vi "Jump To Label.vi"(4 "error in (no error)":errorcluster, 5 "Loop Count (1)":i32=1 min=1 max=65535, 6 "Label  (1)":i32=1 min=1 max=100, 7 "VISA resource name":refnum<visa-resource-name>) -> (0 "error out":errorcluster, 3 "VISA resource name out":refnum<visa-resource-name>)   [LabVIEW 2018, in "Newport ESP301.lvlib"]
doc: "This command changes the flow of the program execution by jumping to a\npredefined label xx. This a flow control command that alters the normal sequential flow of a program. It must be used in conjunction with the DL command which defines a label.\nParameter Loop Count determines the number of times to repeat the jump before allowing the program to flow passed."
uses:
  Newport ESP301.lvlib
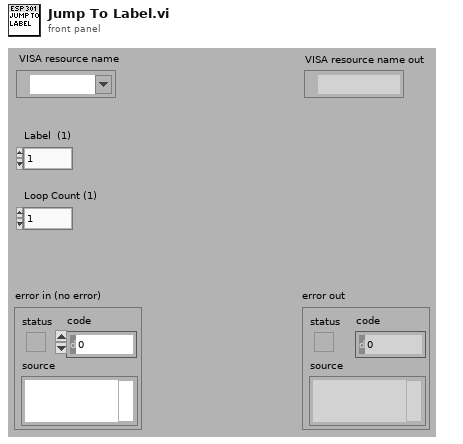
[diagram p1: front panel]
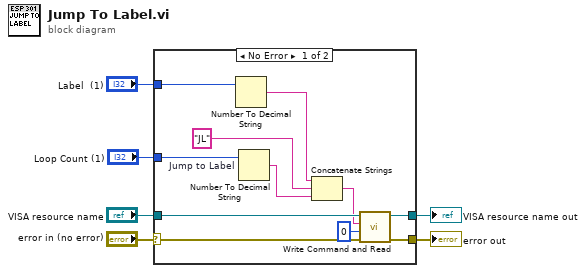
[diagram p0: block diagram]
diagram:
  n1 = case shown="No Error" "error in (no error)" {
    selector: "error in (no error)" -> [w16 w19]
    tunnel: [w15 w19] -> w6
    tunnel: "VISA resource name" -> [w17 w18]
    tunnel: [w14 w18] -> w5
    tunnel: "Label  (1)" -> [w11 _]
    tunnel: "Loop Count (1)" -> [w8 _]
    frame No Error {
      w12 = "JL"  # Jump to Label
      n2 = Number To Decimal String(number=w11) -> (decimal integer string=w13:string)  [unwired: 1 out]
      n3 = Number To Decimal String(number=w8) -> (decimal integer string=w7:string)  [unwired: 1 out]
      n4 = Concatenate Strings(w13, w12, w7) -> (w10:string)
      n5 = call "Write Command and Read.vi"("error in (no error)"=w16, "Bytes to read (100)"=u32 0, "Command"=w10, "VISA resource name"=w17) -> ("error out"=w15:errorcluster, "VISA resource name out"=w14:refnum<visa-resource-name>)  [unwired: 1 in, 3 out]
    }
    frame Error {
    }
  }
  "error out" <- w6
  "VISA resource name out" <- w5
